vi "Output 信息提取.vi"(10 "输出控制":T1) -> (2 "Output 信息配置":string[](array[string]))   [LabVIEW 2017]
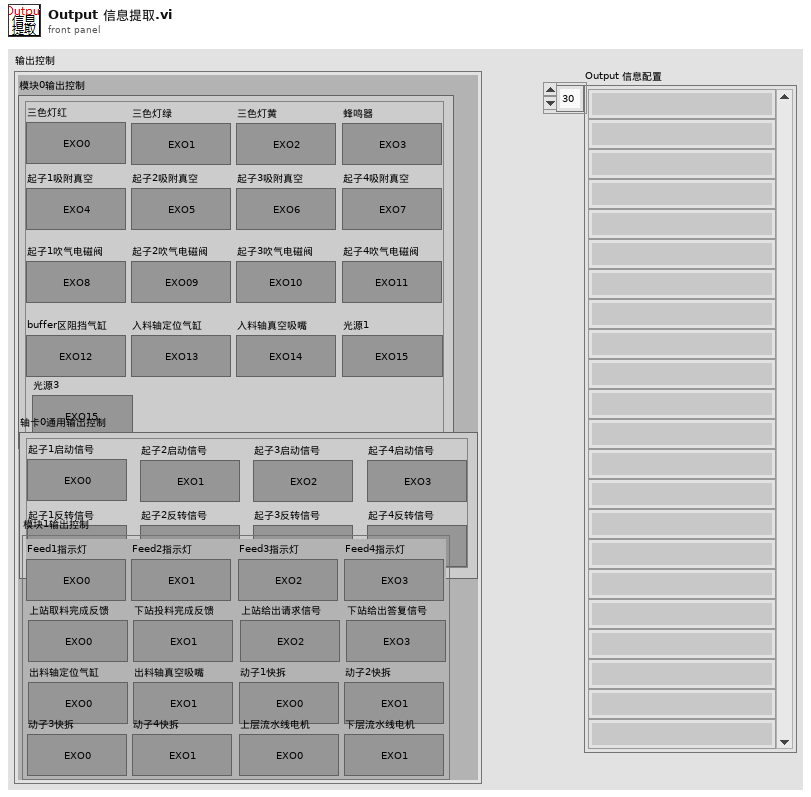
[diagram p1: front panel]
types:
  T1 = typedef "输出控制.ctl" = cluster{"模块0输出控制":T2, "轴卡0通用输出控制":T3, "模块1输出控制":T4}
  T2 = typedef "模块0输出控制.ctl" = cluster{"三色灯红":bool, "三色灯绿":bool, "三色灯黄":bool, "蜂鸣器":bool, "起子1吸附真空":bool, "起子2吸附真空":bool, "起子3吸附真空":bool, "起子4吸附真空":bool, "起子1吹气电磁阀":bool, "起子2吹气电磁阀":bool, "起子3吹气电磁阀":bool, "起子4吹气电磁阀":bool, "buffer区阻挡气缸":bool, "入料轴定位气缸":bool, "入料轴真空吸嘴":bool, "光源1":bool, "光源3":bool}
  T3 = typedef "轴卡0通用输出控制.ctl" = cluster{"起子1启动信号":bool, "起子2启动信号":bool, "起子3启动信号":bool, "起子4启动信号":bool, "起子1反转信号":bool, "起子2反转信号":bool, "起子3反转信号":bool, "起子4反转信号":bool}
  T4 = typedef "模块1输出控制.ctl" = cluster{"Feed1指示灯":bool, "Feed2指示灯":bool, "Feed3指示灯":bool, "Feed4指示灯":bool, "上站取料完成反馈":bool, "下站投料完成反馈":bool, "上站给出请求信号":bool, "下站给出答复信号":bool, "出料轴定位气缸":bool, "出料轴真空吸嘴":bool, "动子1快拆":bool, "动子2快拆":bool, "动子3快拆":bool, "动子4快拆":bool, "上层流水线电机":bool, "下层流水线电机":bool}
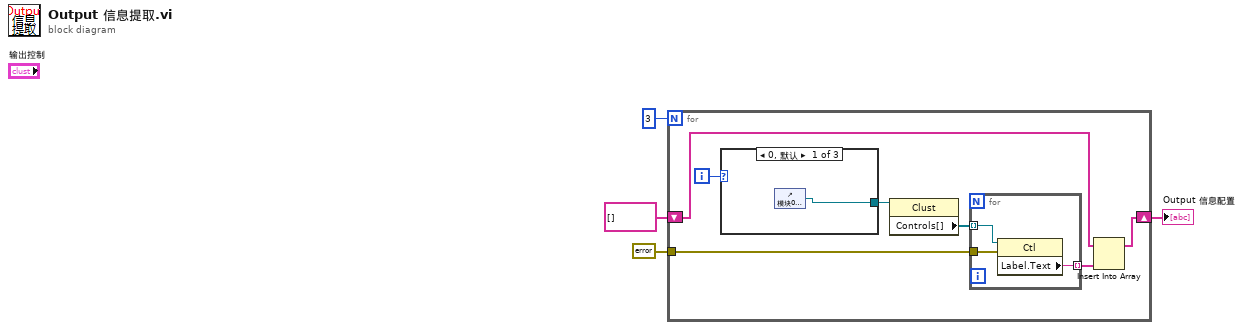
[diagram p0: block diagram]
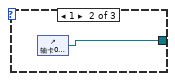
[diagram p2: hidden frame]
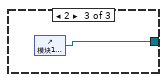
[diagram p3: hidden frame]
diagram:
  n1 = for {
    N: 3 -> [_]
    tunnel: errorcluster {"status"=FALSE, "code"=0, "source"=""} ("错误输入（无错误）") -> [w8]
    shift-right: [w5] -> w1
    shift-left: string[] [] -> [w7]
    i -> [w11]
    n2 = case shown="0, 默认" w11 {
      tunnel: [w15 w16 w17] -> w10
      frame 0, Default {
        n3 = control-ref of="模块0输出控制"() -> (w15:refnum<vi>)
      }
      frame 1 {
        n4 = control-ref of="轴卡0通用输出控制"() -> (w16:refnum<vi>)
      }
      frame 2 {
        n5 = control-ref of="模块1输出控制"() -> (w17:refnum<vi>)
      }
    }
    n6 = property class="Clust"(reference=w10) -> ("Controls[]"=w9:refnum<vi>[])  [unwired: 1 in, 2 out]
    n7 = for {
      tunnel: w9 -> [w14] mode=indexing
      tunnel: w8 -> [w13]
      tunnel: [w12] -> w6 mode=indexing
      n8 = property class="Ctl"(reference=w14, error in=w13) -> ("Label.Text"=w12:string)  [unwired: 2 out]
    }
    n9 = Insert Into Array(array=w7, new element=w6) -> (w5:string[])  [unwired: 1 in]
  }
  "Output 信息配置" <- w1
